vi "touchFromDribblerContact.vi"(8 "error in (no error)":errorcluster, 10 "Game":refnum<class "Game.lvclass">, 11 "Events in":refnum<class "Events.lvclass">) -> (0 "error out":errorcluster, 1 "ballPossession":T1, 2 "touch":bool, 3 "Events out":refnum<class "Events.lvclass">)   [LabVIEW 2023, in "Events.lvclass"]
uses:
  Events.lvclass
  Game_class/Game.lvclass
  Possession.ctl
  Game_class/Game.lvclass/Game.ctl
  Team_class/Team.lvclass/Team.ctl
  Robot_class/Robot.lvclass/Robot.ctl
  RobotFeedback/RobotFeedback.lvclass/RobotFeedback.ctl
  Events.lvclass/Events.ctl
  Write touch.vi
  Write our_balll_possesion.vi
  Write id_touch.vi
  Write id_our_balll_possesion.vi
  Robot_class/Read id.vi
  RobotFeedback/Read dribblerContactToBall.vi
  Game_class/Read AllyRef.vi
  Game_class/Read RobotsFeedback.vi
  Game_class/Read Parameters.lvclass.vi
  Team_class/Read RobotRef.vi
  Read id_touch.vi
  Read id_enemy_ball_possesion.vi
  Read id_our_balll_possesion.vi
  Ally_class/Ally.lvclass
  C:/Users/ebert/Documents/codes/SSL/repo/SSL_AI/Team_class/Team.lvclass
  RobotFeedback/RobotFeedback.lvclass
  Parameters_class/Parameters.lvclass
  Robot_class/Robot.lvclass
  Utilities_class/Utilities.lvclass
panel:
  out "id_our_balll_possesion":i32
  out "id_enemy_ball_possesion":i32
  out "id_touch":i32
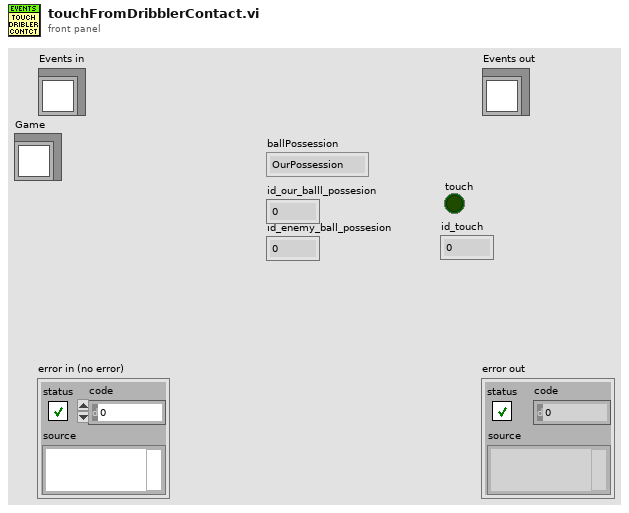
[diagram p1: front panel]
types:
  T1 = typedef "Possession.ctl" = enum16{"OurPossession", "TheirPossession", "Contended", "Loose"}
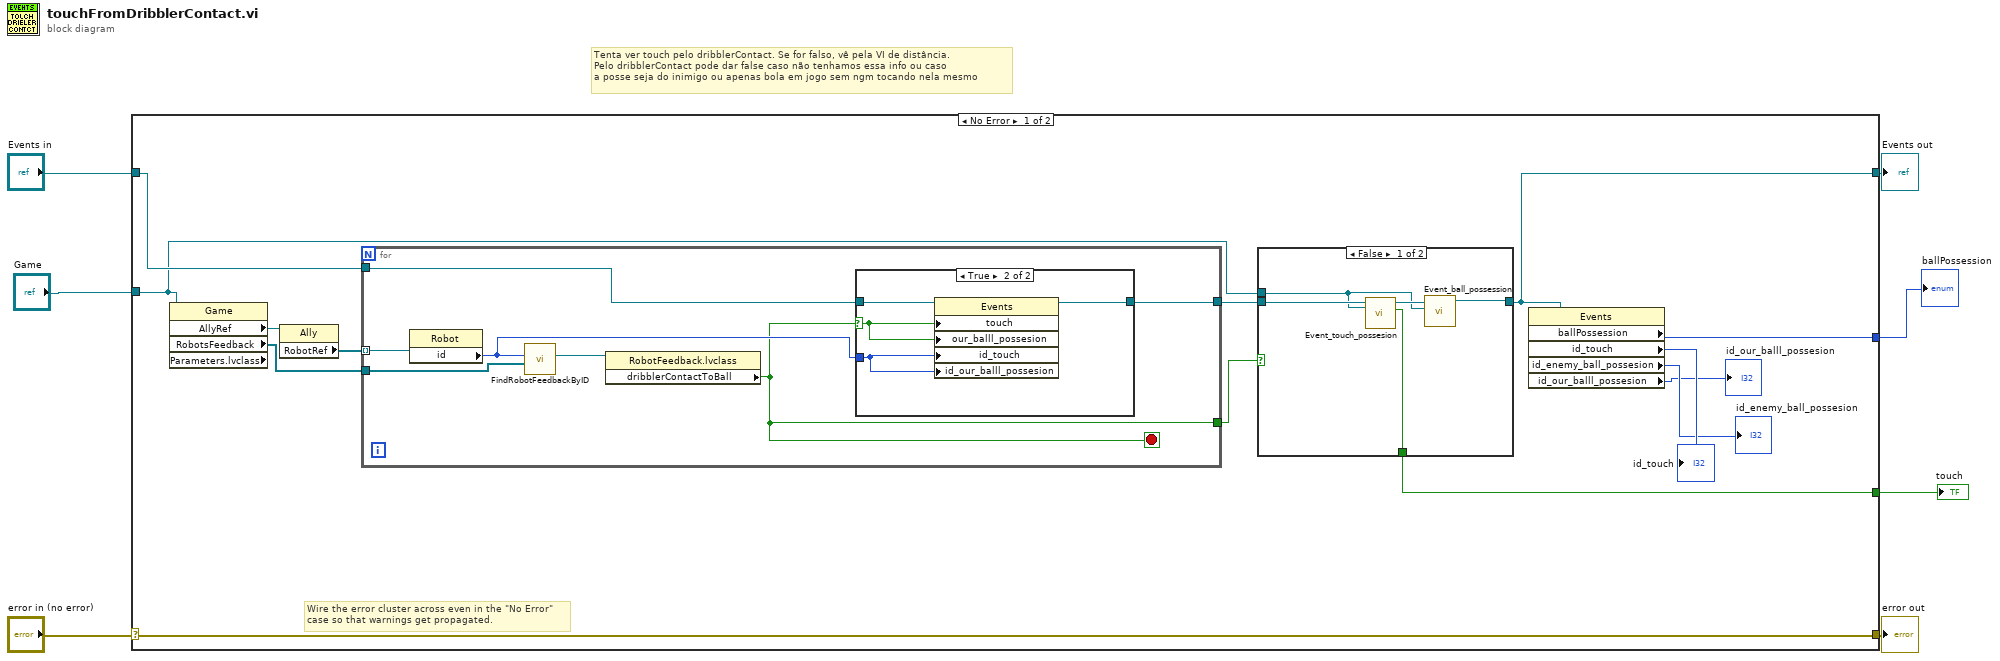
[diagram p0: block diagram]
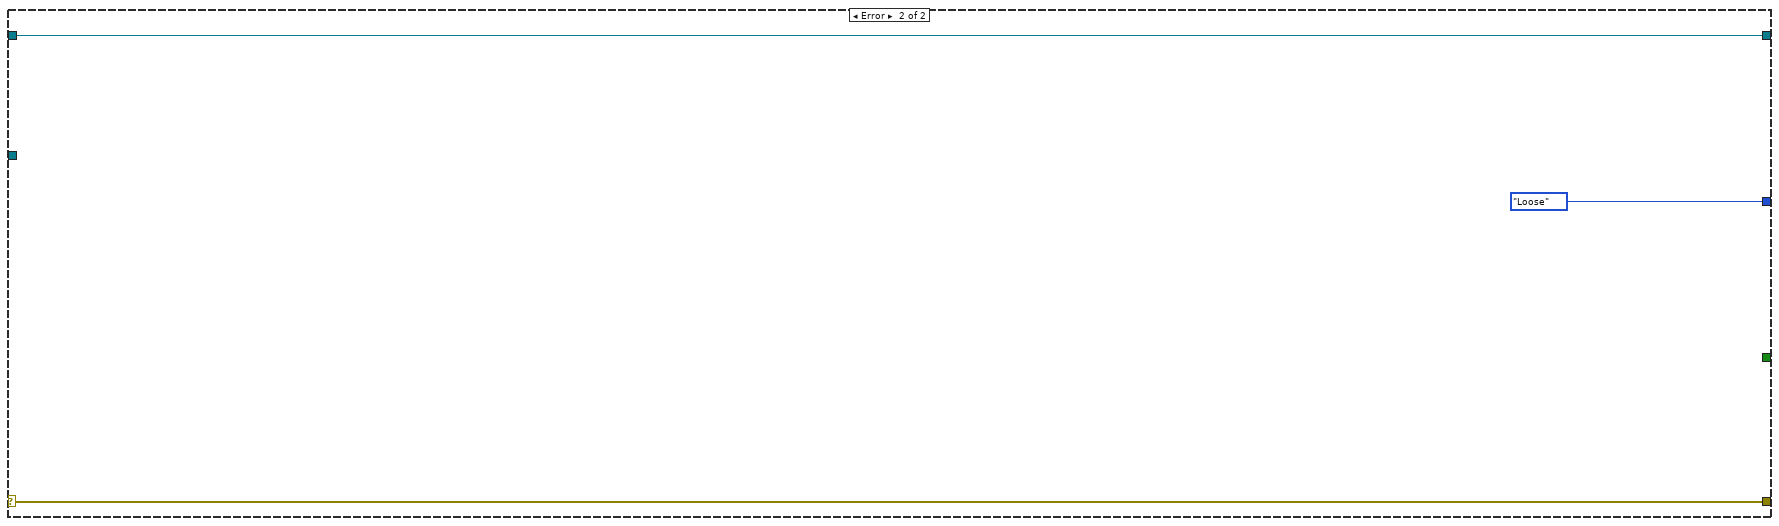
[diagram p4: hidden frame]
diagram:
  # "Tenta ver touch pelo dribblerContact. Se for falso, vê pela VI de distância.\nPelo dribblerContact pode dar false caso não tenhamos essa info ou caso\na posse seja do inimigo ou apenas bola em jogo sem ngm tocando nela mesmo"
  n1 = case shown="No Error" "error in (no error)" {
    selector: "error in (no error)" -> [w21 w43]
    tunnel: [w21 w43] -> w6
    tunnel: [w12 w42] -> w4
    tunnel: "Events in" -> [w17 w42]
    tunnel: "Game" -> [w14 _]
    tunnel: [w13 _] -> w2
    tunnel: [w11 Possession."Loose" ("ballPossession")] -> w1
    frame No Error {
      # "Wire the error cluster across even in the \"No Error\"\ncase so that warnings get propagated."
      n2 = property class="Game" props=["AllyRef", "RobotsFeedback", "Parameters.lvclass"](reference=w14) -> ("AllyRef"=w20:refnum<class "Ally.lvclass">, "RobotsFeedback"=w18:refnum<class "RobotFeedback.lvclass">[])  [unwired: 1 in, 3 out]
      n3 = property class="Ally"(reference=w20) -> ("RobotRef"=w19:refnum<class "Robot.lvclass">[])  [unwired: 1 in, 2 out]
      n4 = for {
        tunnel: w19 -> [w35] mode=indexing
        tunnel: w18 -> [w34]
        tunnel: w17 -> [w32]
        tunnel: [w30] -> w16
        tunnel: [w29] -> w15
        stop <- w30 stop-if-true
        n5 = property class="Robot"(reference=w35) -> ("id"=w31:i32)  [unwired: 1 in, 2 out]
        n6 = call "FindRobotFeedbackByID.vi"("RobotsFeedback"=w34, "id"=w31) -> ("RobotFeedback.lvclass"=w33:refnum<class "RobotFeedback.lvclass">)  [unwired: 6 in, 3 out]
        n7 = property class="RobotFeedback.lvclass"(reference=w33) -> ("dribblerContactToBall"=w30:bool)  [unwired: 1 in, 2 out]
        n8 = case shown="True" w30 {
          selector: w30 -> [_ w39]
          tunnel: w32 -> [w36 w40]
          tunnel: w31 -> [_ w38]
          tunnel: [w36 w37] -> w29
          frame False {
          }
          frame True {
            n9 = property class="Events"(reference=w40, "touch"=w39, "our_balll_possesion"=w39, "id_touch"=w38, "id_our_balll_possesion"=w38) -> (reference out=w37:refnum<class "Events.lvclass">)  [unwired: 1 in, 1 out]
          }
        }
      }
      n10 = case shown="False" w16 {
        selector: w16 -> [_ w27]
        tunnel: w15 -> [w26 w28]
        tunnel: [w23 w28] -> w12
        tunnel: w14 -> [w22 _]
        tunnel: [w25 w27] -> w13
        frame False {
          n11 = call-dynamic "Event_touch_possesion.vi"("Game in"=w22, "Events in"=w26) -> ("touch"=w25:bool, "Events out"=w24:refnum<class "Events.lvclass">)  [unwired: 7 in, 1 out]
          n12 = call-dynamic "Event_ball_possession.vi"("Game 2"=w22, "Events in"=w24) -> ("Events out"=w23:refnum<class "Events.lvclass">)  [unwired: 8 in, 1 out]
        }
        frame True {
        }
      }
      n13 = property class="Events"(reference=w12) -> ("ballPossession"=w11:T1, "id_touch"=→"id_touch":i32, "id_enemy_ball_possesion"=→"id_enemy_ball_possesion":i32, "id_our_balll_possesion"=→"id_our_balll_possesion":i32)  [unwired: 1 in, 2 out]
    }
    frame Error {
    }
  }
  "error out" <- w6
  "Events out" <- w4
  "touch" <- w2
  "ballPossession" <- w1
